vi "helper-eng-clock-src.vi"(10 "Clk Simulator":timestamp, 11 "Time Addition":dbl) -> (1 "Time Stamp":timestamp, 2 "Clk Simulated":bool, 3 "CLK":dbl format="%#.0f")   [LabVIEW 2024]
panel:
  out "clk":dbl
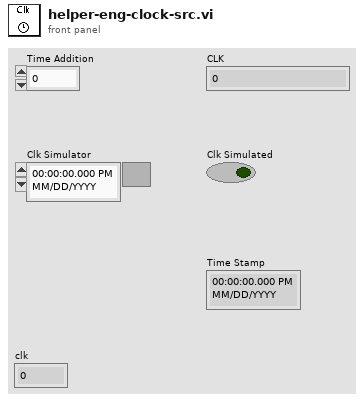
[diagram p1: front panel]
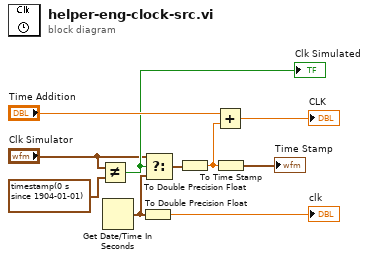
[diagram p0: block diagram]
diagram:
  n1 = Not Equal?(x="Clk Simulator", y=timestamp(0 s since 1904-01-01)) -> (x != y?=w4:bool)
  "Clk Simulated" <- w4
  n2 = Get Date/Time In Seconds() -> (seconds since 1Jan1904=w2:timestamp)
  n3 = To Double Precision Float(number=w2) -> (double precision float=→"clk":dbl)
  n4 = Select(t="Clk Simulator", s=w4, f=w2) -> (s? t:f=w6:timestamp)
  n5 = To Double Precision Float(number=w6) -> (double precision float=w9:dbl)
  n6 = Add(x="Time Addition", y=w9) -> (x+y=→"CLK":dbl)
  n7 = To Time Stamp(1:w9) -> (0:→"Time Stamp":timestamp)
